vi "hse-application_SetFrameworkVersion.vi"(8 "error in":errorcluster, 11 "Framework Version Number":string) -> (0 "error out":errorcluster)   [LabVIEW 2020, in "hse-application.lvclass"]
doc: "Stores the version number of the framework for later usage (display, logging, ...).\n\n\n\n____\nHAMPEL SOFTWARE ENGINEERING v3.8.0 (2023-12-18 14:41)"
uses:
  hse-application.lvclass
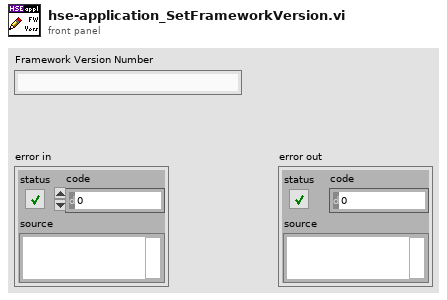
[diagram p1: front panel]
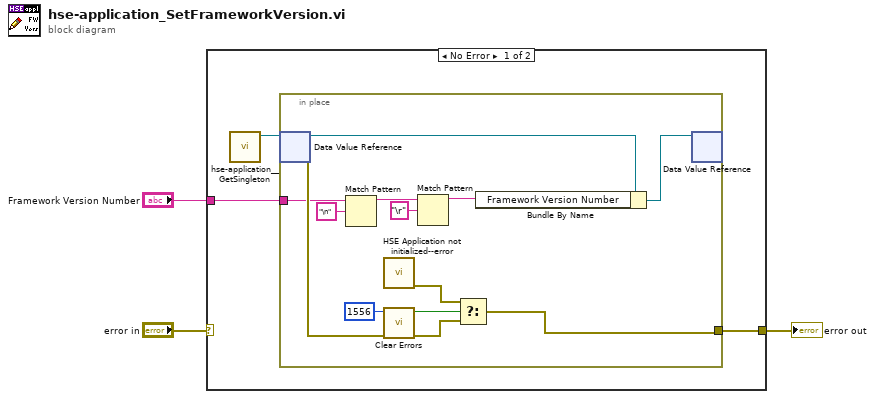
[diagram p0: block diagram]
diagram:
  n1 = case shown="No Error" "error in" {
    selector: "error in" -> [_ w20]
    tunnel: [w6 w20] -> w2
    tunnel: "Framework Version Number" -> [w4 _]
    frame No Error {
      n2 = call "hse-application__GetSingleton.vi"() -> ("ApplicationClass DVR"=w5:refnum<data-value>)  [unwired: 10 in, 1 out]
      n3 = in-place "In Place Element Structure" {
        in-place-border: [w16] -> w6
        in-place-border: w4 -> [w10]
        n4 = in-place-dvr #1(w5) -> (w15:refnum<class "hse-application.lvclass">, w17:errorcluster)
        n5 = Match Pattern(string=w10, regular expression="\n") -> (before substring=w13:string)  [unwired: 1 in, 3 out]
        n6 = call "HSE Application not initialized--error.vi"() -> ("error out"=w19:errorcluster)  [unwired: 11 in]
        n7 = call <vilib>:"Clear Errors.vi"("error in (no error)"=w17, "specific error code to clear (0: all)"=1556) -> ("error out"=w18:errorcluster, "specific error cleared?"=w7:bool)  [unwired: 4 in]
        n8 = Match Pattern(string=w13, regular expression="\r") -> (before substring=w9:string)  [unwired: 1 in, 3 out]
        n9 = Select(t=w19, s=w7, f=w18) -> (s? t:f=w16:errorcluster)
        n10 = Bundle By Name(cluster=w15, "Framework Version Number"=w9) -> (w14:refnum<class "hse-application.lvclass">)
        n11 = in-place-dvr #1(w14) -> ()  [unwired: 2 out]
      }
    }
    frame Error {
    }
  }
  "error out" <- w2
